vi "goto room.vi"(8 "error in (no error)":errorcluster, 9 "Position":T1, 11 "main.ctl":T2) -> (0 "error out":errorcluster, 1 "Position out":T1)   [LabVIEW 2019]
uses:
  main data.ctl
  vision/vision_board_ctl.ctl
  block box.ctl
  subVI/move/position cluster.ctl
  route_name.ctl
panel:
  out "room":string[](array[string])
  out "Color":string[](array[string])
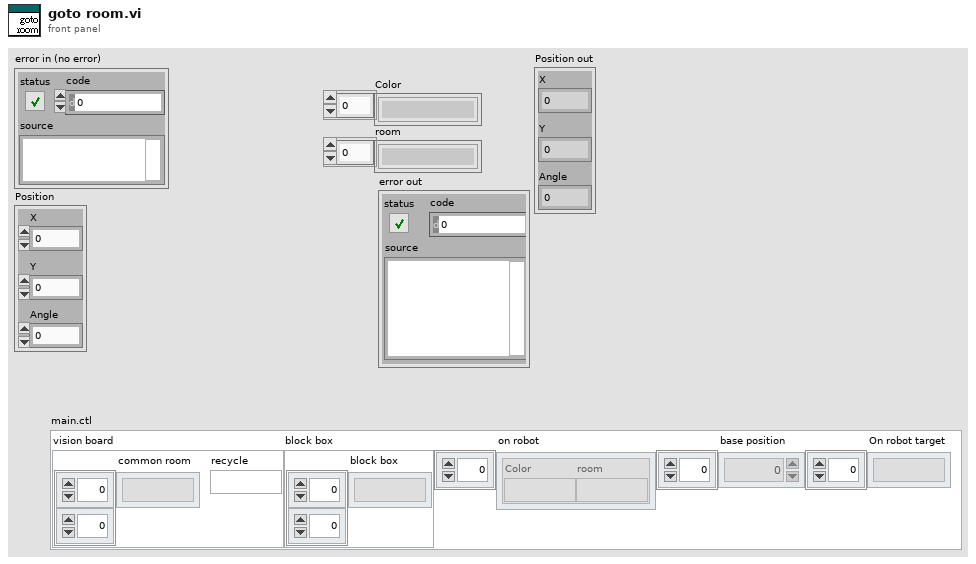
[diagram p1: front panel]
types:
  T1 = typedef "position cluster.ctl" = cluster{"X":dbl, "Y":dbl, "Angle":dbl}
  T2 = typedef "main data.ctl" = cluster{"vision board":T3, "block box":T4, "on robot ":cluster{"Color":string, "room":string}[], "base position":dbl[], "On robot target":string[]}
  T3 = typedef "vision_board_ctl.ctl" = cluster{"common room":string[][], "recycle":string}
  T4 = typedef "block box.ctl" = cluster{"block box":string[][]}
  T5 = typedef "route_name.ctl" = enum16{"S-Vision", "Vision-R1", "Vision-R2", "Vision-R3", "Vision-R4", "Vision-R5", "R1-Vision", "R2-Vision", "R3-Vision", "R4-Vision", "R5-Vision", "Vision-box", "box-recycle", "recycle-box", "box-Vision", "Vision-S"}
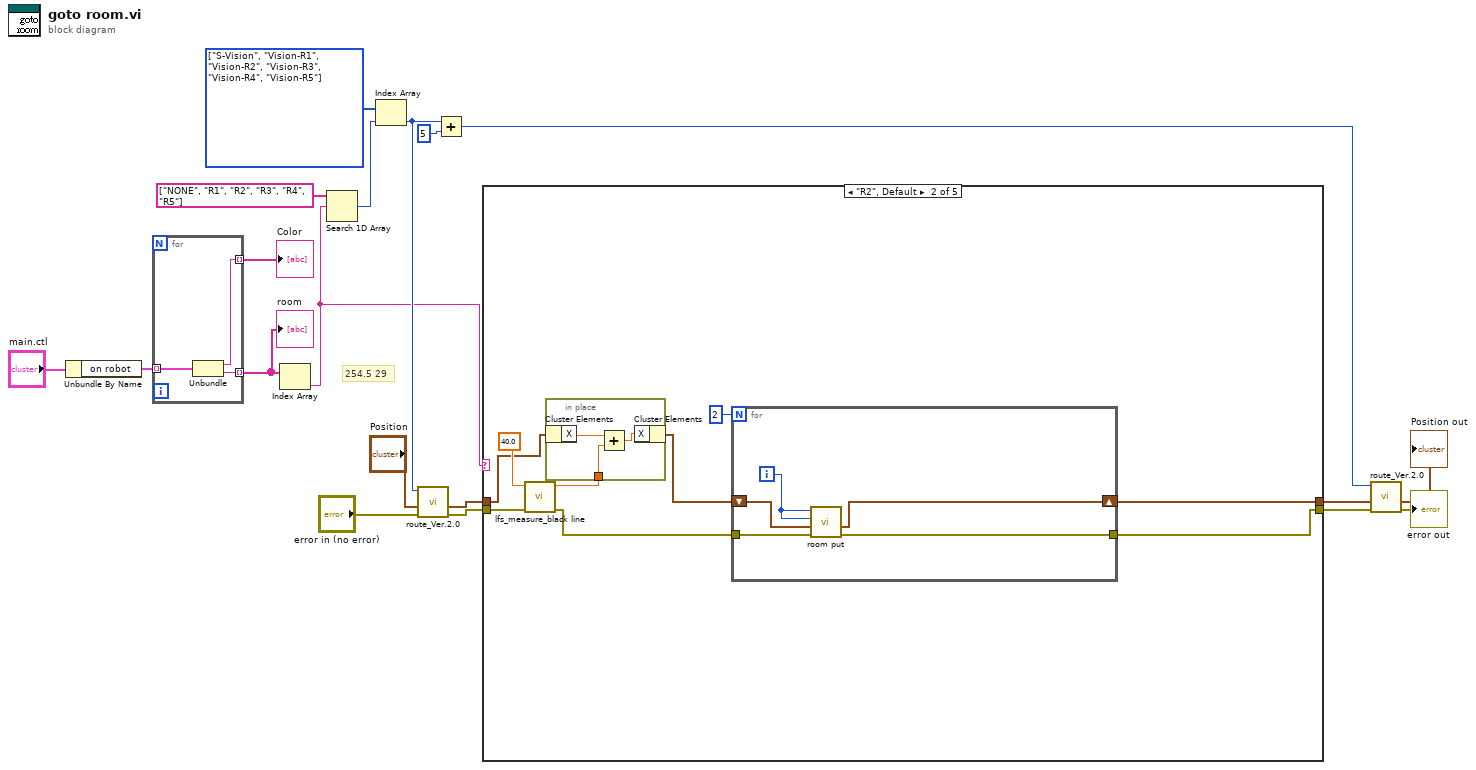
[diagram p0: block diagram]
diagram:
  w14 = T5[] [enum."S-Vision", enum."Vision-R1", enum."Vision-R2", enum."Vision-R3", enum."Vision-R4", enum."Vision-R5"] items=["S-Vision", "Vision-R1", "Vision-R2", "Vision-R3", "Vision-R4", "Vision-R5", "R1-Vision", "R2-Vision", "R3-Vision", "R4-Vision", "R5-Vision", "Vision-box", "box-recycle", "recycle-box", "box-Vision", "Vision-S"]
  # "254.5 29"
  n1 = Unbundle By Name("main.ctl") -> ("on robot"=w18:cluster{"Color":string, "room":string}[])
  n2 = for {
    tunnel: w18 -> [w22] mode=indexing
    tunnel: [w21] -> w17 mode=indexing
    tunnel: [w20] -> w16 mode=indexing
    n3 = Unbundle(w22) -> ("Color"=w21:string, "room"=w20:string)
  }
  "Color" <- w17
  "room" <- w16
  n4 = Index Array(array=w16) -> (element=w7:string)  [unwired: 1 in]
  n5 = Search 1D Array(1D array=string[] ["NONE", "R1", "R2", "R3", "R4", "R5"], element=w7) -> (index of element=w13:i32)  [unwired: 1 in]
  n6 = Index Array(array=w14, index=w13) -> (element=w12:T5)
  n7 = call "route_Ver.2.0.vi"("error in (no error)"="error in (no error)", "Position"="Position", 11:w12) -> ("error out"=w9:errorcluster, "Position out"=w8:T1)  [unwired: 7 in]
  n8 = Add(x=w12, y=5) -> (x+y=w10:i32)
  n9 = case shown="\"R2\", Default" w7 {
    tunnel: w9 -> [w23 w33 w42 w44 w46]
    tunnel: w8 -> [w24 w31 w43 w45 w47]
    tunnel: [w24 w27 w43 w45 w47] -> w6
    tunnel: [w23 w26 w42 w44 w46] -> w5
    frame "R1" {
    }
    frame "R2", Default {
      n10 = call "lfs_measure_black line.vi"("error in (no error)"=w33, "limit"=40.0) -> ("error out"=w25:errorcluster, "move cm"=w30:dbl)  [unwired: 7 in, 1 out]
      n11 = in-place {
        in-place-border: w30 -> [w39]
        n12 = in-place-cluster #1(w31) -> ("X"=w41:dbl)
        n13 = Add(x=w41, y=w39) -> (x+y=w40:dbl)
        n14 = in-place-cluster #1("X"=w40) -> (w28:T1)
      }
      n15 = for {
        N: 2 -> [_]
        tunnel: [w35] -> w26
        shift-right: [w36] -> w27
        shift-left: w28 -> [w37]
        tunnel: w25 -> [w34]
        i -> [w38]
        n16 = call "room put.vi"("error in (no error)"=w34, "Position in"=w37, "register address"=w38, "put layer"=w38) -> ("error out"=w35:errorcluster, "Position out"=w36:T1)  [unwired: 6 in]
      }
    }
    frame "R3" {
    }
    frame "R4" {
    }
    frame "R5" {
    }
  }
  n17 = call "route_Ver.2.0.vi"("error in (no error)"=w5, "Position"=w6, 11:w10) -> ("error out"=→"error out":errorcluster, "Position out"=→"Position out":T1)  [unwired: 7 in]
